vi "testDMA_9040(chunk).vi"() -> ()   [LabVIEW 2020]
uses:
  <vilib>/rvi/Emulation/niFpgaGetClockAttributes.vi
  <vilib>/rvi/Emulation/niFpgaSctlEmulationGetInTimedLoop.vi
  <vilib>/rvi/Emulation/niFpgaEmulationReportErrorSimple.vi
  <vilib>/rvi/DataTransferAndStorage/Container/Common/niFpgaContainerExecOnDevCompGetState.vi
  <vilib>/rvi/Emulation/niFpgaEmulationIsFPGAContextNoSignature.vi
  <vilib>/rvi/errors/niFpgaSetErrorForExecOnDevCompSimple.vi
  <vilib>/rvi/eio/common/nirviEmuReportErrorAndStop.vi
  <vilib>/rvi/DataTransferAndStorage/Container/Common/niFpgaContainerGetUniqueNameForEmu.vi
  <vilib>/rvi/FIFO/Fifo_Resource/nirvififoEmulationSetSize.vi
  <vilib>/rvi/FIFO/Fifo_Resource/nirviFifoEmulationQueueMgr.vi
  <instcachedir>/0/nirviFifoEmulationQueueMgr_E5CAEC123FF24DC58D834DCA3CDAA9B5.lvgen/nirviFifoEmulationQueueMgr_E5CAEC123FF24DC58D834DCA3CDAA9B5_001.vi
  <vilib>/rvi/FIFO/Fifo_Resource/nirvififoEmulationDetermineInputValidOut.vi
  <vilib>/rvi/FIFO/Fifo_Resource/nirvififoEmulationCreateLock.vi
  <vilib>/rvi/Emulation/niFpgaProcessEmulError.vi
  <vilib>/rvi/FIFO/Fifo_Resource/nirvififoEmulationObtainLock.vi
  <vilib>/rvi/FIFO/Fifo_Resource/nirvififoEmulationReleaseLock.vi
  <vilib>/rvi/occurrence/nirviWaitOnOccurrenceBase.vi
  <vilib>/rvi/errors/nirviReportUnexpectedCaseInternalError.vi
  <vilib>/rvi/errors/nirviReportUnexpectedCaseInternalError (U32).vi
  <vilib>/Utility/error.llb/Clear Errors.vi
  <vilib>/rvi/interface/RandomDataEmulation/niFpgaRandomDataHandleErrors.vi
  <vilib>/rvi/Emulation/niFpgaCriticalErrorInLSC.vi
  <vilib>/rvi/DataTransferAndStorage/Container/XNode/niFpgaContainer.xnode
  <vilib>/rvi/FIFO/Fifo_Resource/niFpgaFifoEmulationRefIn.vi
panel:
  out "write DMA timeout count 2":i16
  out "dma read time ticks 2":u32
  out "dma read time ticks":u32
  out "write DMA timeout count":i16
  in  "number of samples":i16=100
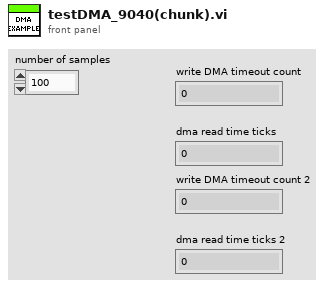
[diagram p1: front panel]
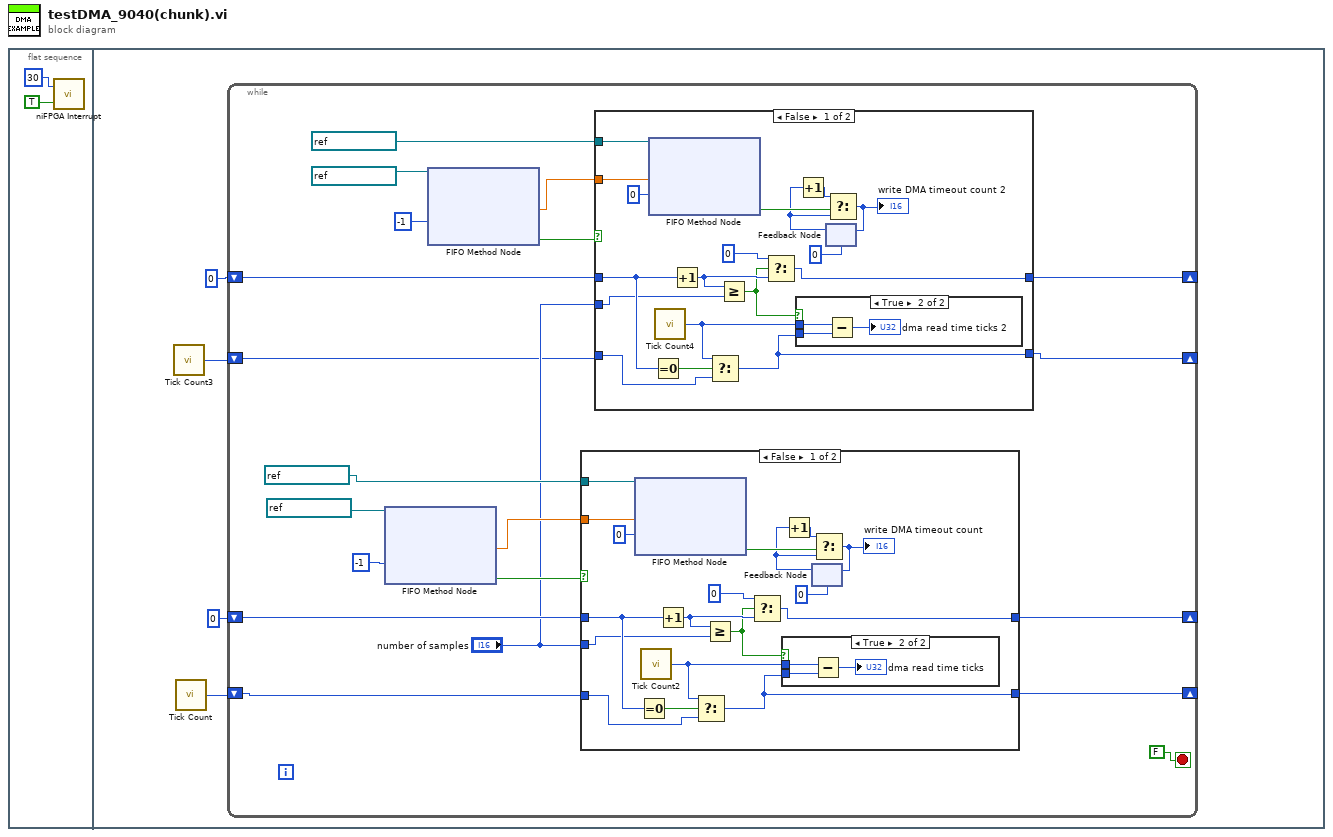
[diagram p0: block diagram]
diagram:
  n1 = flat-sequence {
    frame #0 {
      n2 = call <vilib>:"niFPGA Interrupt.vi"("Wait Until Cleared (F)"=TRUE, "IRQ Number (0)"=u8 30) -> ()  [unwired: 1 in]
    }
    frame #1 {
      n3 = call "Tick Count3"() -> ("Tick Count(Ticks)"=w4:u32)
      n4 = call "Tick Count"() -> ("Tick Count(Ticks)"=w5:u32)
      n5 = while {
        shift-right: [w18] -> _
        shift-left: i16 0 -> [w20]
        shift-right: [w17] -> _
        shift-left: w5 -> [w19]
        shift-right: [w8] -> _
        shift-left: i16 0 -> [w11]
        shift-right: [w7] -> _
        shift-left: w4 -> [w9]
        stop <- FALSE stop-if-true
        n6 = xnode ("FIFO Method Node")("Timeout"=-1, "FIFO In"=refnum<k21> "Incoming1") -> ("Element"=w25:sgl, "Timed Out?"=w21:bool)  [unwired: 1 out]
        n7 = xnode ("FIFO Method Node")("Timeout"=-1, "FIFO In"=refnum<k21> "Incoming2") -> ("Element"=w14:sgl, "Timed Out?"=w13:bool)  [unwired: 1 out]
        n8 = case shown="False" w21 {
          tunnel: refnum<k21> "Outgoing1" ("FIFO In") -> [w67 _]
          tunnel: w25 -> [w66 _]
          tunnel: w20 -> [w58 w72]
          tunnel: "number of samples" -> [w57 _]
          tunnel: w19 -> [w53 w71]
          tunnel: [w54 w72] -> w18
          tunnel: [w50 w71] -> w17
          frame False {
            n9 = xnode ("FIFO Method Node")("Element"=w66, "Timeout"=0, "FIFO In"=w67) -> ("Timed Out?"=w65:bool)  [unwired: 1 out]
            n10 = Equal To 0?(x=w58) -> (x = 0?=w59:bool)
            n11 = call "Tick Count2"() -> ("Tick Count(Ticks)"=w51:u32)
            n12 = Increment(x=w58) -> (x+1=w55:i16)
            n13 = Select(t=w51, s=w59, f=w53) -> (s? t:f=w50:u32)
            n14 = Greater Or Equal?(x=w55, y=w57) -> (x >= y?=w52:bool)
            n15 = Select(t=i16 0, s=w52, f=w55) -> (s? t:f=w54:i16)
            n16 = case shown="True" w52 {
              tunnel: w51 -> [_ w69]
              tunnel: w50 -> [_ w70]
              frame False {
              }
              frame True {
                n17 = Subtract(x=w69, y=w70) -> (x-y=→"dma read time ticks":u32)
              }
            }
            n18 = feedback #1(i16 0) -> (w63:i16)
            n19 = Increment(x=w63) -> (x+1=w62:i16)
            n20 = Select(t=w62, s=w65, f=w63) -> (s? t:f=w61:i16)
            "write DMA timeout count" <- w61
            n21 = feedback-in #1(w61) -> ()
          }
          frame True {
          }
        }
        n22 = case shown="False" w13 {
          tunnel: refnum<k21> "Outgoing2" ("FIFO In") -> [w44 _]
          tunnel: w14 -> [w43 _]
          tunnel: w11 -> [w35 w49]
          tunnel: "number of samples" -> [w34 _]
          tunnel: w9 -> [w30 w48]
          tunnel: [w31 w49] -> w8
          tunnel: [w27 w48] -> w7
          frame False {
            n23 = xnode ("FIFO Method Node")("Element"=w43, "Timeout"=0, "FIFO In"=w44) -> ("Timed Out?"=w42:bool)  [unwired: 1 out]
            n24 = Equal To 0?(x=w35) -> (x = 0?=w36:bool)
            n25 = call "Tick Count4"() -> ("Tick Count(Ticks)"=w28:u32)
            n26 = Increment(x=w35) -> (x+1=w32:i16)
            n27 = Select(t=w28, s=w36, f=w30) -> (s? t:f=w27:u32)
            n28 = Greater Or Equal?(x=w32, y=w34) -> (x >= y?=w29:bool)
            n29 = Select(t=i16 0, s=w29, f=w32) -> (s? t:f=w31:i16)
            n30 = case shown="True" w29 {
              tunnel: w28 -> [_ w46]
              tunnel: w27 -> [_ w47]
              frame False {
              }
              frame True {
                n31 = Subtract(x=w46, y=w47) -> (x-y=→"dma read time ticks 2":u32)
              }
            }
            n32 = feedback #2(i16 0) -> (w40:i16)
            n33 = Increment(x=w40) -> (x+1=w39:i16)
            n34 = Select(t=w39, s=w42, f=w40) -> (s? t:f=w38:i16)
            "write DMA timeout count 2" <- w38
            n35 = feedback-in #2(w38) -> ()
          }
          frame True {
          }
        }
      }
    }
  }
